vi "TelnetClient4.vi"(4 "Input Command 2":string="P15=1", 5 "IP Address":string="192.168.0.103", 6 "Input Command":string="P15=0", 7 "Port #":i32=1000) -> (0 "Telnet error":errorcluster, 1 "Command and Results":string, 2 "Command and Results 2":string, 3 "Open Connection":string)   [LabVIEW 2013]
doc: "The Telnet Line Client VI uses the Telnet VIs to simulate a simple Telnet Window."
uses:
  <vilib>/addons/internet/NI_InternetTK_Core_VIs.lvlib
panel:
  # "Netburner Telnet Reset Routine"
  # "(Pxx = 0 or 1, to set line xx true or false. Reset is active low)"
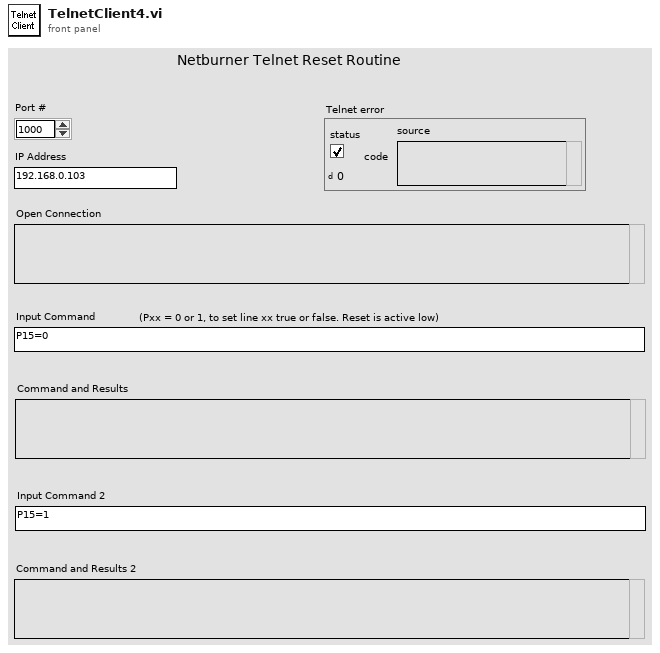
[diagram p1: front panel]
types:
  T1 = typedef "Telnet Session.ctl" = refnum<k1>
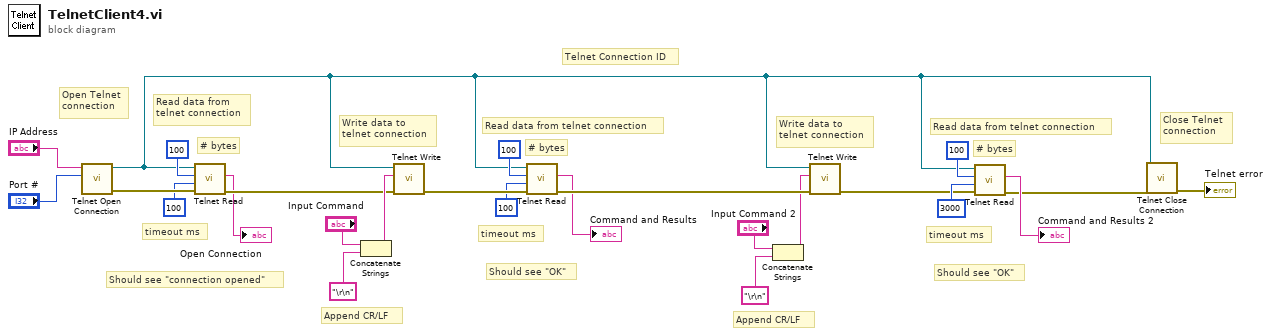
[diagram p0: block diagram]
diagram:
  # "timeout ms"
  # "# bytes"
  # "Should see \"OK\""
  # "Read data from telnet connection"
  # "timeout ms"
  # "# bytes"
  # "Should see \"OK\""
  # "Read data from telnet connection"
  # "Write data to \ntelnet connection"
  # "Append CR/LF"
  # "Append CR/LF"
  # "Telnet Connection ID"
  # "timeout ms"
  # "# bytes"
  # "Should see \"connection opened\""
  # "Write data to \ntelnet connection"
  # "Read data from \ntelnet connection"
  # "Close Telnet \nconnection"
  # "Open Telnet\nconnection"
  n1 = call <vilib>:"Telnet Open Connection.vi"("remote port (23)"="Port #", "address"="IP Address") -> ("error out"=w23:errorcluster, "telnet connection"=w3:T1)  [unwired: 2 in, 6 out]
  n2 = call <vilib>:"Telnet Read.vi"("error in (no error)"=w23, "timeout ms (25000)"=100, "bytes to read"=100, "telnet connection"=w3) -> ("error out"=w17:errorcluster, "data out"=→"Open Connection":string)  [unwired: 4 out]
  n3 = Concatenate Strings("Input Command", "\r\n") -> (w18:string)
  n4 = call <vilib>:"Telnet Write.vi"("error in (no error)"=w17, "data in"=w18, "telnet connection"=w3) -> ("error out"=w16:errorcluster)  [unwired: 1 in, 5 out]
  n5 = call <vilib>:"Telnet Read.vi"("error in (no error)"=w16, "timeout ms (25000)"=100, "bytes to read"=100, "telnet connection"=w3) -> ("error out"=w13:errorcluster, "data out"=→"Command and Results":string)  [unwired: 4 out]
  n6 = Concatenate Strings("Input Command 2", "\r\n") -> (w10:string)
  n7 = call <vilib>:"Telnet Write.vi"("error in (no error)"=w13, "data in"=w10, "telnet connection"=w3) -> ("error out"=w2:errorcluster)  [unwired: 1 in, 5 out]
  n8 = call <vilib>:"Telnet Read.vi"("error in (no error)"=w2, "timeout ms (25000)"=3000, "bytes to read"=100, "telnet connection"=w3) -> ("error out"=w1:errorcluster, "data out"=→"Command and Results 2":string)  [unwired: 4 out]
  n9 = call <vilib>:"Telnet Close Connection.vi"("error in (no error)"=w1, "telnet connection"=w3) -> ("error out"=→"Telnet error":errorcluster)  [unwired: 9 out]
